vi "IMAQ FPGA Camera Link Data to Pixels 1 Tap 16-Bit.vi"(1 "Camera Link Data":cluster{"Port A":u8, "Port B":u8}) -> (0 "Pixel":u16)   [LabVIEW 2017]
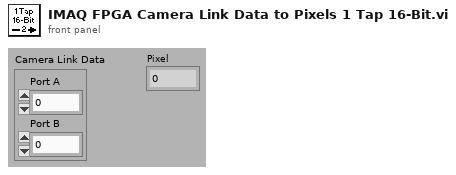
[diagram p1: front panel]
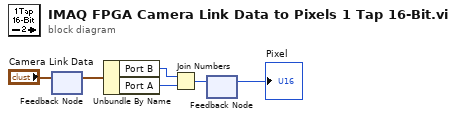
[diagram p0: block diagram]
diagram:
  n1 = feedback #1() -> (w1:cluster{"Port A":u8, "Port B":u8})  [unwired: 1 in]
  n2 = feedback-in #1("Camera Link Data") -> ()
  n3 = Unbundle By Name(w1) -> ("Port B"=w5:u8, "Port A"=w4:u8)
  n4 = Join Numbers(hi=w5, lo=w4) -> ((hi.lo)=w6:u16)
  n5 = feedback-in #2(w6) -> ()
  n6 = feedback #2() -> (→"Pixel":u16)  [unwired: 1 in]
